vi "Construct Listbox Bus Monitor Panel.vi"(10 "Show Panel Boolean":string) -> (3 "ListboxBusMonitorPanel out":refnum<class "ListboxBusMonitorPanel.lvclass">)   [LabVIEW 2020, in "ListboxBusMonitor.lvlib" / "ListboxBusMonitorPanel.lvclass"]
uses:
  <vilib>/gpm_packages/@cs/BusMonitor/ListboxBusMonitor/ListboxBusMonitorPanel/ListboxBusMonitorPanel.lvclass
  <vilib>/gpm_packages/@cs/BusMonitor/ListboxBusMonitor/ListboxBusMonitorPanel/ListboxBusMonitorPanel.lvclass/ListboxBusMonitorPanel.ctl
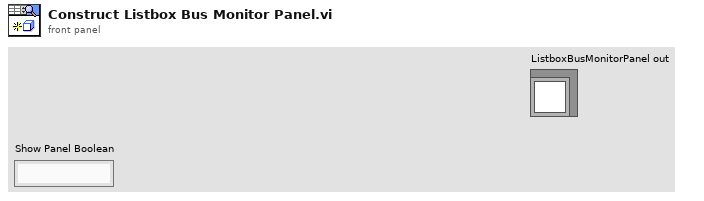
[diagram p1: front panel]
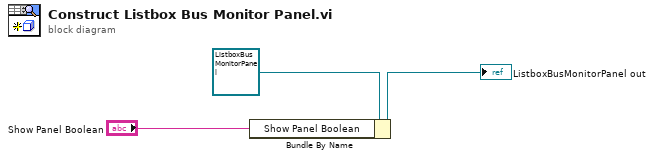
[diagram p0: block diagram]
diagram:
  n1 = Bundle By Name(cluster=refnum<class "ListboxBusMonitorPanel.lvclass"> refnum ("ListboxBusMonitorPanel in"), "Show Panel Boolean"="Show Panel Boolean") -> (→"ListboxBusMonitorPanel out":refnum<class "ListboxBusMonitorPanel.lvclass">)
